vi "powerLaserOff.vi"(8 "error in (no error)":errorcluster, 11 "Parser in":refnum<class "CommandCreator.lvclass">) -> (0 "error out":errorcluster, 2 "command":string, 3 "Parser out":refnum<class "CommandCreator.lvclass">)   [LabVIEW 2016, in "CommandCreator.lvclass"]
uses:
  CommandCreator.lvclass
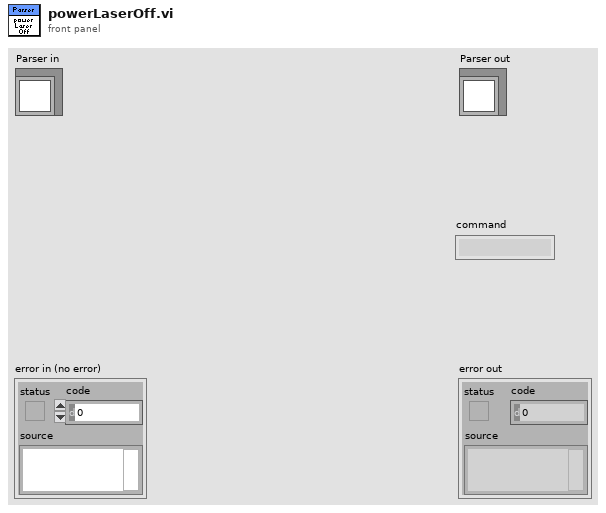
[diagram p1: front panel]
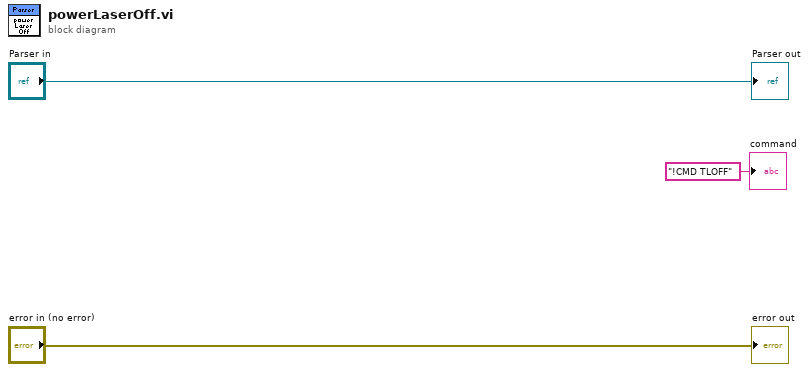
[diagram p0: block diagram]
diagram:
  "error out" <- "error in (no error)"
  "Parser out" <- "Parser in"
  "command" <- "!CMD TLOFF" ("command")
